vi "登陆界面.vi"() -> ()   [LabVIEW 2018]
panel:
  in  "密码":string
  in  "账号":string
  in  "注册账号vi路径":path=path "E:/登陆系统重写/注册账号.vi"
  in  "添加按钮":bool
  in  "密码路径":path=path "E:/登陆系统重写/密码.txt"
  in  "账户路径":path=path "E:/登陆系统重写/账户.txt"
  in  "VI路径":path=path "E:/登陆系统重写/癌变与普通病变选择界面.vi"
  in  "登录按钮":bool
  # "AI智能辅助内镜诊断病变软件系统"
  # "用户登录"
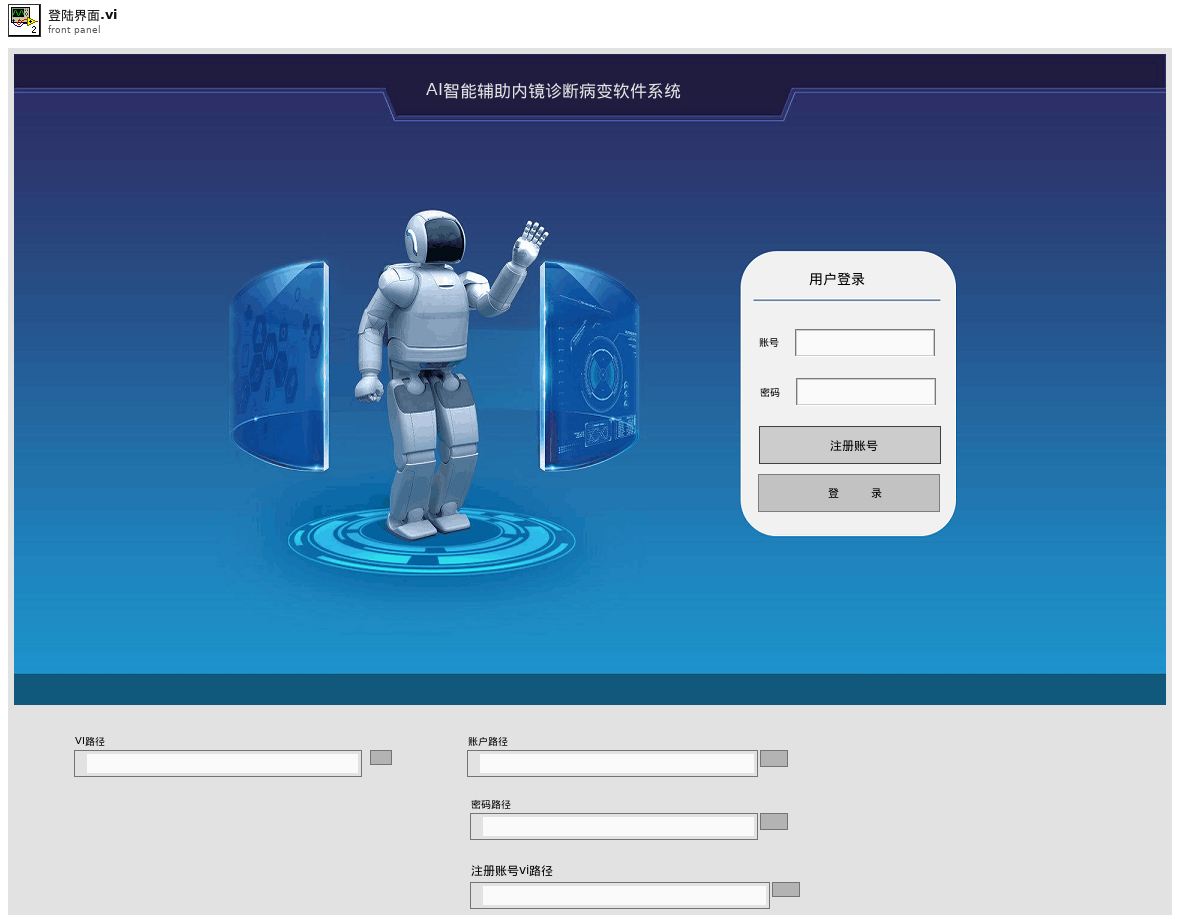
[diagram p1: front panel]
types:
  T1 = enum32{"Invalid", "Standard", "Closed", "Hidden", "Minimized", "Maximized"}
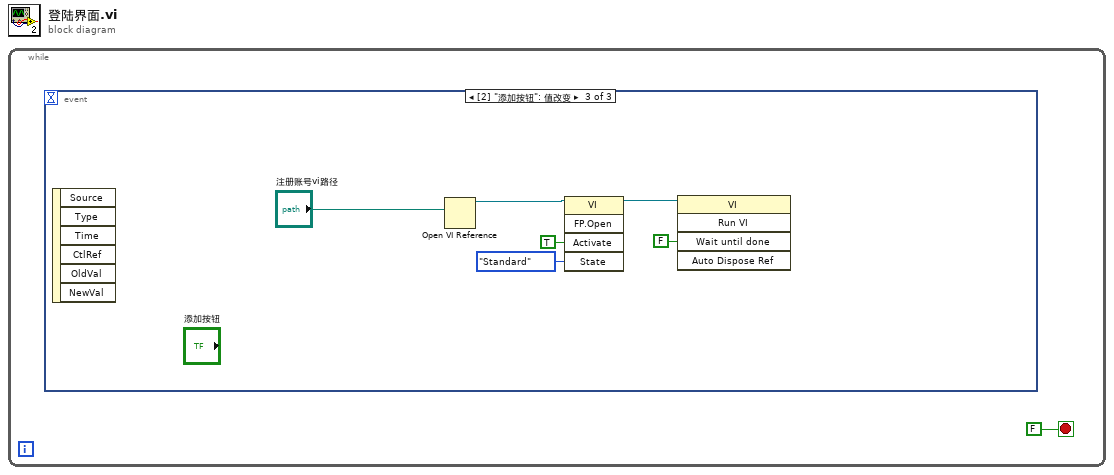
[diagram p0: block diagram]
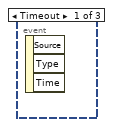
[diagram p2: hidden frame]
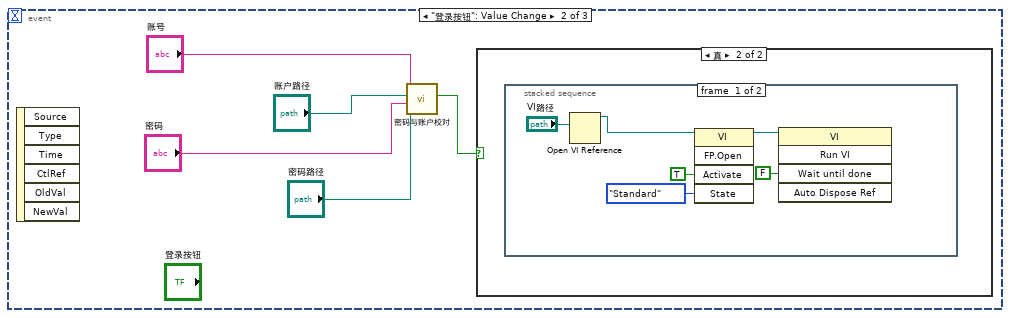
[diagram p3: hidden frame]
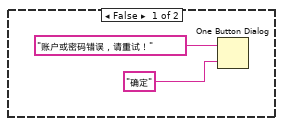
[diagram p4: hidden frame]
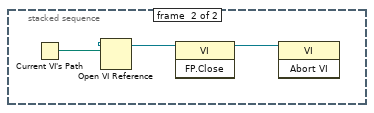
[diagram p5: hidden frame]
diagram:
  n1 = while {
    stop <- FALSE stop-if-true
    n2 = event shown="[2] \"添加按钮\": 值改变" {
      selector: _ -> [_ _ _]
      dyn-events: _ -> [_ _ _]
      timeout: _ -> [_ _ _]
      event Timeout {
        n3 = event-data() -> ()  [unwired: 1 in, 3 out]
      }
      event "登录按钮": Value Change {
        n4 = event-data() -> ()  [unwired: 1 in, 6 out]
        n5 = call "密码与账户校对.vi"("密码路径"="密码路径", "密码"="密码", "账户路径"="账户路径", "账户"="账号") -> ("x与y？"=w6:bool)  [unwired: 7 in]
        n6 = case shown="真" w6 {
          frame False {
            n7 = One Button Dialog(message="账户或密码错误，请重试！" ("消息"), button name ("OK")="确定" ("按钮名称（“确定”）")) -> ()  [unwired: 1 out]
          }
          frame True {
            n8 = stacked-sequence {
              frame #0 {
                n9 = Open VI Reference(vi path="VI路径") -> (vi reference=w13:refnum<vi>)  [unwired: 5 in, 1 out]
                n10 = invoke class="VI" method="FP.Open"(reference=w13, "Activate"=TRUE ("激活？"), "State"=T1."Standard" ("状态")) -> (reference out=w12:refnum<vi>)  [unwired: 2 in, 4 out]
                n11 = invoke class="VI" method="Run VI"(reference=w12, "Wait until done"=FALSE ("结束前等待")) -> ()  [unwired: 3 in, 5 out]
              }
              frame #1 {
                n12 = Current VI's Path() -> (path=w17:path)
                n13 = Open VI Reference(vi path=w17) -> (vi reference=w16:refnum<vi>)  [unwired: 5 in, 1 out]
                n14 = invoke class="VI" method="FP.Close"(reference=w16) -> (reference out=w15:refnum<vi>)  [unwired: 2 in, 2 out]
                n15 = invoke class="VI" method="Abort VI"(reference=w15) -> ()  [unwired: 2 in, 3 out]
              }
            }
          }
        }
      }
      event "添加按钮": Value Change {
        n16 = event-data() -> ()  [unwired: 1 in, 6 out]
        n17 = Open VI Reference(vi path="注册账号vi路径") -> (vi reference=w22:refnum<vi>)  [unwired: 5 in, 1 out]
        n18 = invoke class="VI" method="FP.Open"(reference=w22, "Activate"=TRUE ("激活？"), "State"=T1."Standard" ("状态")) -> (reference out=w19:refnum<vi>)  [unwired: 2 in, 4 out]
        n19 = invoke class="VI" method="Run VI"(reference=w19, "Wait until done"=FALSE ("结束前等待")) -> ()  [unwired: 3 in, 5 out]
      }
    }
  }
